vi "Lab Panel V4.90.vi"() -> ()   [LabVIEW 2013] (continued)
                    n844 = local read "SIG LAB04-1"() -> (w1524:T2)
                    n845 = stacked-sequence {
                      seq-local: [w1535 _] -> [_ w1539]
                      tunnel: w1533 -> [_ w1549]
                      tunnel: w1532 -> [_ w1548]
                      tunnel: w1531 -> [_ w1547]
                      tunnel: w1530 -> [_ w1546]
                      tunnel: w1529 -> [_ w1545]
                      tunnel: [_ w1544] -> w1528
                      tunnel: w1527 -> [_ w1543]
                      tunnel: w1526 -> [_ w1542]
                      tunnel: w1525 -> [_ w1541]
                      tunnel: w1524 -> [w1534 w1540]
                      tunnel: w1523 -> [_ w1538]
                      frame #0 {
                        n846 = Unbundle(w1534) -> ("AMPS"=w1537:dbl)  [unwired: 4 out]
                        n847 = call "Check For Amps on v1.vi"("ID"="LAB04-1", "amps"=w1537) -> ("amps"=w1535:bool)  [unwired: 9 in]
                      }
                      frame #1 {
                        n848 = case shown="True" w1539 {
                          tunnel: w1549 -> [_ w1562]
                          tunnel: w1548 -> [_ w1561]
                          tunnel: w1547 -> [_ w1560]
                          tunnel: w1546 -> [_ w1559]
                          tunnel: w1545 -> [_ w1558]
                          tunnel: [errorcluster {"status"=FALSE, "code"=0, "source"=""} ("error out") w1557] -> w1544
                          tunnel: w1543 -> [_ w1556]
                          tunnel: w1542 -> [_ w1555]
                          tunnel: w1541 -> [_ w1554]
                          tunnel: w1540 -> [_ w1553]
                          tunnel: w1538 -> [_ w1552]
                          frame False {
                            w1550 = FALSE
                            n849 = local write "RUN LAB04-1"(w1550) -> ()
                            n850 = local write "run lab04-1"(w1550) -> ()
                          }
                          frame True {
                            n851 = stacked-sequence {
                              seq-local: [w1563 _ _ _ _] -> [_ w1587 _ _ _]
                              tunnel: w1562 -> [w1568 _ _ _ _]
                              tunnel: w1561 -> [w1564 _ _ _ _]
                              tunnel: w1560 -> [w1578 _ _ _ _]
                              tunnel: w1559 -> [w1571 _ _ _ _]
                              tunnel: w1558 -> [w1566 _ _ _ _]
                              tunnel: [_ w1582 _ _ _] -> w1557
                              tunnel: w1556 -> [_ _ _ w1608 _]
                              tunnel: w1555 -> [_ _ _ w1607 _]
                              tunnel: w1554 -> [_ _ _ w1606 _]
                              tunnel: w1553 -> [_ _ _ _ _]
                              tunnel: w1552 -> [_ _ _ _ w1622]
                              frame #0 {
                                w1565 = "\\"
                                n852 = local read "SET LAB04-1"() -> (w1573:T5)
                                n853 = case shown="\"CYCLE TEST\"" w1578 {
                                tunnel: ["L04-1-CHART TEST-" "L04-1-CYCLE TEST-" "L04-1-T-RISE TEST-"] -> w1574
                                frame "CHART TEST", Default {
                                }
                                frame "CYCLE TEST" {
                                }
                                frame "T-RISE TEST" {
                                }
                                }
                                n854 = Unbundle(w1573) -> ("DESCRIPTION"=w1572:string)  [unwired: 4 out]
                                n855 = Concatenate Strings(w1568, "\\", w1566, w1565, w1564, w1565) -> (w1575:string)
                                n856 = String To Path(string=w1575) -> (path=w1577:path)
                                n857 = Concatenate Strings(w1575, w1574, w1572, "-", w1571, ".tdms") -> (w1563:string)
                                n858 = Create Folder(path (use dialog)=w1577) -> (error out=w1576:errorcluster)  [unwired: 2 in, 2 out]
                                n859 = global write "Global 1.vi" "LAB04-1 FILE"(w1563) -> ()
                                n860 = call <vilib>:"Clear Errors.vi"("error in (no error)"=w1576) -> ()  [unwired: 6 in, 1 out]
                              }
                              frame #1 {
                                (unwired) FALSE
                                n861 = String To Path(string=w1587) -> (path=w1583:path)
                                n862 = TDMS Open(6:FALSE, 10:T20."create or replace" ("operation (0:open)"), 11:w1583) -> (0:w1582:errorcluster, 3:→"TDMS LAB04-1":refnum<k34>)  [unwired: 4 in]
                              }
                              frame #2 {
                                n863 = local read "SET LAB04-1"() -> (w1593:T5)
                                n864 = local read "TDMS LAB04-1"() -> (w1604:refnum<k34>)
                                n865 = Build Array("Testers Name", "Description", "Set Test Cycles", "T-Rise minutes", "T-Rise Deg C") -> (w1594:string[])
                                n866 = Unbundle(w1593) -> ("NAME"=w1592:string, "DESCRIPTION"=w1591:string, "CYCLES"=w1590:dbl, "T-RISE mins"=w1589:dbl, "T-RISE deg C"=w1588:dbl)
                                n867 = Number To Decimal String(number=w1590) -> (decimal integer string=w1603:string)  [unwired: 1 in]
                                n868 = Number To Decimal String(number=w1589) -> (decimal integer string=w1602:string)  [unwired: 1 in]
                                n869 = Number To Decimal String(number=w1588) -> (decimal integer string=w1601:string)  [unwired: 1 in]
                                n870 = Build Array(w1592, w1591, w1603, w1602, w1601) -> (w1600:string[])
                                n871 = TDMS Set Properties(5:w1600, 7:w1594, 11:w1604) -> ()  [unwired: 3 in, 4 out]
                              }
                              frame #3 {
                                n872 = local read "DISP LAB04-1"() -> (w1609:T4)
                                n873 = Concatenate Strings("LAB04-1  ", w1608) -> (w1610:string)
                                n874 = Two Button Dialog(message=w1610, 1:w1606, 2:w1607) -> (T button?=w1612:bool)
                                n875 = case shown="True" w1612 {
                                tunnel: w1609 -> [w1619 w1620]
                                tunnel: [w1619 w1620] -> w1616
                                tunnel: [w1618 w1621] -> w1615
                                tunnel: [w1617 w1621] -> w1614
                                frame False {
                                n876 = Unbundle(w1619) -> ("CYCLE"=w1618:dbl, "MINS"=w1617:dbl)  [unwired: 1 out]
                                }
                                frame True {
                                w1621 = 0.0
                                }
                                }
                                n877 = Bundle(cluster=w1616, "CYCLE"=w1615, "MINS"=w1614, "STATUS"="RUN") -> (w1605:T4)
                                n878 = local write "DISP LAB04-1"(w1605) -> ()
                              }
                              frame #4 {
                                n879 = local read "TEMP START LAB04-1"() -> (w1624:cluster{"TL":dbl, "TN":dbl})
                                n880 = Bundle(cluster=w1624, "TL"=w1622, "TN"=w1622) -> (w1623:cluster{"TL":dbl, "TN":dbl})
                                n881 = local write "TEMP START LAB04-1"(w1623) -> ()
                              }
                            }
                          }
                        }
                      }
                    }
                  }
                }
              }
              event "RUN LAB04-2": Value Change {
                n882 = event-data() -> ("NewVal"=w1629:bool)  [unwired: 1 in, 5 out]
                n883 = local write "run lab04-2"(w1629) -> ()
                n884 = case shown="True" w1629 {
                  tunnel: w1635 -> [_ w1673]
                  tunnel: w1634 -> [_ w1672]
                  tunnel: w1632 -> [w1637 w1671]
                  tunnel: w1633 -> [_ w1670]
                  tunnel: w1631 -> [_ w1669]
                  tunnel: [w1636 w1668] -> w1630
                  tunnel: w1628 -> [_ w1667]
                  tunnel: w1627 -> [_ w1666]
                  tunnel: w1626 -> [_ w1665]
                  tunnel: w1625 -> [_ w1663]
                  frame False {
                    # "stop test"
                    n885 = stacked-sequence {
                      tunnel: w1637 -> [w1646 _]
                      tunnel: [w1638 _] -> w1636
                      frame #0 {
                        n886 = local read "DISP LAB04-2"() -> (w1645:T4)
                        n887 = Unbundle(w1645) -> ("CYCLE"=w1643:dbl, "MINS"=w1644:dbl)  [unwired: 1 out]
                        n888 = case shown="\"CYCLE TEST\"" w1646 {
                          tunnel: w1644 -> [_ _ w1653]
                          tunnel: w1643 -> [w1651 w1652 _]
                          tunnel: [w1651 w1652 w1653] -> w1642
                          frame "CHART TEST", Default {
                          }
                          frame "CYCLE TEST" {
                          }
                          frame "T-RISE TEST" {
                          }
                        }
                        n889 = local read "TDMS LAB04-2"() -> (w1650:refnum<k34>)
                        n890 = Build Array("STOPPED") -> (w1647:string[])
                        n891 = Build Array(w1642) -> (w1641:dbl[])
                        n892 = TDMS Write(0:w1650, 5:"TEST RESULT", 7:w1647, 9:w1641) -> (4:w1639:refnum<k34>, 15:w1640:errorcluster)  [unwired: 2 in, 2 out]
                        n893 = TDMS Close(8:w1640, 11:w1639) -> (0:w1638:errorcluster)  [unwired: 1 out]
                      }
                      frame #1 {
                        n894 = local read "DISP LAB04-2"() -> (w1657:T4)
                        n895 = stacked-sequence {
                          tunnel: "LAB04-2" -> [w1659 w1661]
                          frame #0 {
                            n896 = call "sub vi - defrag tdms v1.vi"("panel id"=w1659) -> ("error out"=w1658:errorcluster)  [unwired: 10 in]
                            n897 = local write "data file error"(w1658) -> ()
                          }
                          frame #1 {
                            n898 = call "Save data file (stop) v3.vi"("panel id"=w1661) -> ("network file save error"=w1660:errorcluster)  [unwired: 9 in, 1 out]
                            n899 = local write "RESULT LAB04-2"(FALSE) -> ()
                            n900 = local write "data file error"(w1660) -> ()
                          }
                        }
                        n901 = Bundle(cluster=w1657, "STATUS"="STOP") -> (w1655:T4)  [unwired: 2 in]
                        n902 = local write "DISP LAB04-2"(w1655) -> ()
                      }
                    }
                  }
                  frame True {
                    n903 = local read "SIG LAB04-2"() -> (w1664:T2)
                    n904 = stacked-sequence {
                      seq-local: [w1675 _] -> [_ w1679]
                      tunnel: w1673 -> [_ w1689]
                      tunnel: w1672 -> [_ w1688]
                      tunnel: w1671 -> [_ w1687]
                      tunnel: w1670 -> [_ w1686]
                      tunnel: w1669 -> [_ w1685]
                      tunnel: [_ w1684] -> w1668
                      tunnel: w1667 -> [_ w1683]
                      tunnel: w1666 -> [_ w1682]
                      tunnel: w1665 -> [_ w1681]
                      tunnel: w1664 -> [w1674 w1680]
                      tunnel: w1663 -> [_ w1678]
                      frame #0 {
                        n905 = Unbundle(w1674) -> ("AMPS"=w1677:dbl)  [unwired: 4 out]
                        n906 = call "Check For Amps on v1.vi"("ID"="LAB04-2", "amps"=w1677) -> ("amps"=w1675:bool)  [unwired: 9 in]
                      }
                      frame #1 {
                        n907 = case shown="True" w1679 {
                          tunnel: w1689 -> [_ w1702]
                          tunnel: w1688 -> [_ w1701]
                          tunnel: w1687 -> [_ w1700]
                          tunnel: w1686 -> [_ w1699]
                          tunnel: w1685 -> [_ w1698]
                          tunnel: [errorcluster {"status"=FALSE, "code"=0, "source"=""} ("error out") w1697] -> w1684
                          tunnel: w1683 -> [_ w1696]
                          tunnel: w1682 -> [_ w1695]
                          tunnel: w1681 -> [_ w1694]
                          tunnel: w1680 -> [_ w1693]
                          tunnel: w1678 -> [_ w1692]
                          frame False {
                            w1690 = FALSE
                            n908 = local write "RUN LAB04-2"(w1690) -> ()
                            n909 = local write "run lab04-2"(w1690) -> ()
                          }
                          frame True {
                            n910 = stacked-sequence {
                              seq-local: [w1703 _ _ _ _] -> [_ w1727 _ _ _]
                              tunnel: w1702 -> [w1708 _ _ _ _]
                              tunnel: w1701 -> [w1704 _ _ _ _]
                              tunnel: w1700 -> [w1718 _ _ _ _]
                              tunnel: w1699 -> [w1711 _ _ _ _]
                              tunnel: w1698 -> [w1706 _ _ _ _]
                              tunnel: [_ w1722 _ _ _] -> w1697
                              tunnel: w1696 -> [_ _ _ w1748 _]
                              tunnel: w1695 -> [_ _ _ w1747 _]
                              tunnel: w1694 -> [_ _ _ w1746 _]
                              tunnel: w1693 -> [_ _ _ _ _]
                              tunnel: w1692 -> [_ _ _ _ w1762]
                              frame #0 {
                                w1705 = "\\"
                                n911 = local read "SET LAB04-2"() -> (w1713:T5)
                                n912 = case shown="\"CHART TEST\", Default" w1718 {
                                tunnel: ["L04-2-CHART TEST-" "L04-2-CYCLE TEST-" "L04-2-T-RISE TEST-"] -> w1714
                                frame "CHART TEST", Default {
                                }
                                frame "CYCLE TEST" {
                                }
                                frame "T-RISE TEST" {
                                }
                                }
                                n913 = Unbundle(w1713) -> ("DESCRIPTION"=w1712:string)  [unwired: 4 out]
                                n914 = Concatenate Strings(w1708, "\\", w1706, w1705, w1704, w1705) -> (w1715:string)
                                n915 = String To Path(string=w1715) -> (path=w1717:path)
                                n916 = Concatenate Strings(w1715, w1714, w1712, "-", w1711, ".tdms") -> (w1703:string)
                                n917 = Create Folder(path (use dialog)=w1717) -> (error out=w1716:errorcluster)  [unwired: 2 in, 2 out]
                                n918 = global write "Global 1.vi" "LAB04-2 FILE"(w1703) -> ()
                                n919 = call <vilib>:"Clear Errors.vi"("error in (no error)"=w1716) -> ()  [unwired: 6 in, 1 out]
                              }
                              frame #1 {
                                (unwired) FALSE
                                n920 = String To Path(string=w1727) -> (path=w1723:path)
                                n921 = TDMS Open(6:FALSE, 10:T20."create or replace" ("operation (0:open)"), 11:w1723) -> (0:w1722:errorcluster, 3:→"TDMS LAB04-2":refnum<k34>)  [unwired: 4 in]
                              }
                              frame #2 {
                                n922 = local read "SET LAB04-2"() -> (w1733:T5)
                                n923 = local read "TDMS LAB04-2"() -> (w1744:refnum<k34>)
                                n924 = Build Array("Testers Name", "Description", "Set Test Cycles", "T-Rise minutes", "T-Rise Deg C") -> (w1734:string[])
                                n925 = Unbundle(w1733) -> ("NAME"=w1732:string, "DESCRIPTION"=w1731:string, "CYCLES"=w1730:dbl, "T-RISE mins"=w1729:dbl, "T-RISE deg C"=w1728:dbl)
                                n926 = Number To Decimal String(number=w1730) -> (decimal integer string=w1743:string)  [unwired: 1 in]
                                n927 = Number To Decimal String(number=w1729) -> (decimal integer string=w1742:string)  [unwired: 1 in]
                                n928 = Number To Decimal String(number=w1728) -> (decimal integer string=w1741:string)  [unwired: 1 in]
                                n929 = Build Array(w1732, w1731, w1743, w1742, w1741) -> (w1740:string[])
                                n930 = TDMS Set Properties(5:w1740, 7:w1734, 11:w1744) -> ()  [unwired: 3 in, 4 out]
                              }
                              frame #3 {
                                n931 = local read "DISP LAB04-2"() -> (w1749:T4)
                                n932 = Concatenate Strings("LAB04-2 ", w1748) -> (w1750:string)
                                n933 = Two Button Dialog(message=w1750, 1:w1746, 2:w1747) -> (T button?=w1752:bool)
                                n934 = case shown="True" w1752 {
                                tunnel: w1749 -> [w1759 w1760]
                                tunnel: [w1759 w1760] -> w1756
                                tunnel: [w1758 w1761] -> w1755
                                tunnel: [w1757 w1761] -> w1754
                                frame False {
                                n935 = Unbundle(w1759) -> ("CYCLE"=w1758:dbl, "MINS"=w1757:dbl)  [unwired: 1 out]
                                }
                                frame True {
                                w1761 = 0.0
                                }
                                }
                                n936 = Bundle(cluster=w1756, "CYCLE"=w1755, "MINS"=w1754, "STATUS"="RUN") -> (w1745:T4)
                                n937 = local write "DISP LAB04-2"(w1745) -> ()
                              }
                              frame #4 {
                                n938 = local read "TEMP START LAB04-2"() -> (w1764:cluster{"TL":dbl, "TN":dbl})
                                n939 = Bundle(cluster=w1764, "TL"=w1762, "TN"=w1762) -> (w1763:cluster{"TL":dbl, "TN":dbl})
                                n940 = local write "TEMP START LAB04-2"(w1763) -> ()
                              }
                            }
                          }
                        }
                      }
                    }
                  }
                }
              }
              event "RUN LAB05-1": Value Change {
                n941 = event-data() -> ("NewVal"=w1769:bool)  [unwired: 1 in, 5 out]
                n942 = local write "run lab05-1"(w1769) -> ()
                n943 = case shown="True" w1769 {
                  tunnel: w1775 -> [_ w1813]
                  tunnel: w1774 -> [_ w1812]
                  tunnel: w1772 -> [w1777 w1811]
                  tunnel: w1773 -> [_ w1810]
                  tunnel: w1771 -> [_ w1809]
                  tunnel: [w1776 w1808] -> w1770
                  tunnel: w1768 -> [_ w1807]
                  tunnel: w1767 -> [_ w1806]
                  tunnel: w1766 -> [_ w1805]
                  tunnel: w1765 -> [_ w1803]
                  frame False {
                    # "stop test"
                    n944 = stacked-sequence {
                      tunnel: w1777 -> [w1786 _]
                      tunnel: [w1778 _] -> w1776
                      frame #0 {
                        n945 = local read "DISP LAB05-1"() -> (w1785:T4)
                        n946 = Unbundle(w1785) -> ("CYCLE"=w1783:dbl, "MINS"=w1784:dbl)  [unwired: 1 out]
                        n947 = case shown="\"CYCLE TEST\"" w1786 {
                          tunnel: w1784 -> [_ _ w1793]
                          tunnel: w1783 -> [w1791 w1792 _]
                          tunnel: [w1791 w1792 w1793] -> w1782
                          frame "CHART TEST", Default {
                          }
                          frame "CYCLE TEST" {
                          }
                          frame "T-RISE TEST" {
                          }
                        }
                        n948 = local read "TDMS LAB05-1"() -> (w1790:refnum<k34>)
                        n949 = Build Array("STOPPED") -> (w1787:string[])
                        n950 = Build Array(w1782) -> (w1781:dbl[])
                        n951 = TDMS Write(0:w1790, 5:"TEST RESULT", 7:w1787, 9:w1781) -> (4:w1779:refnum<k34>, 15:w1780:errorcluster)  [unwired: 2 in, 2 out]
                        n952 = TDMS Close(8:w1780, 11:w1779) -> (0:w1778:errorcluster)  [unwired: 1 out]
                      }
                      frame #1 {
                        n953 = local read "DISP LAB05-1"() -> (w1797:T4)
                        n954 = stacked-sequence {
                          tunnel: "LAB05-1" -> [w1799 w1801]
                          frame #0 {
                            n955 = call "sub vi - defrag tdms v1.vi"("panel id"=w1799) -> ("error out"=w1798:errorcluster)  [unwired: 10 in]
                            n956 = local write "data file error"(w1798) -> ()
                          }
                          frame #1 {
                            n957 = call "Save data file (stop) v3.vi"("panel id"=w1801) -> ("network file save error"=w1800:errorcluster)  [unwired: 9 in, 1 out]
                            n958 = local write "RESULT LAB05-1"(FALSE) -> ()
                            n959 = local write "data file error"(w1800) -> ()
                          }
                        }
                        n960 = Bundle(cluster=w1797, "STATUS"="STOP") -> (w1795:T4)  [unwired: 2 in]
                        n961 = local write "DISP LAB05-1"(w1795) -> ()
                      }
                    }
                  }
                  frame True {
                    n962 = local read "SIG LAB05-1"() -> (w1804:T2)
                    n963 = stacked-sequence {
                      seq-local: [w1815 _] -> [_ w1819]
                      tunnel: w1813 -> [_ w1829]
                      tunnel: w1812 -> [_ w1828]
                      tunnel: w1811 -> [_ w1827]
                      tunnel: w1810 -> [_ w1826]
                      tunnel: w1809 -> [_ w1825]
                      tunnel: [_ w1824] -> w1808
                      tunnel: w1807 -> [_ w1823]
                      tunnel: w1806 -> [_ w1822]
                      tunnel: w1805 -> [_ w1821]
                      tunnel: w1804 -> [w1814 w1820]
                      tunnel: w1803 -> [_ w1818]
                      frame #0 {
                        n964 = Unbundle(w1814) -> ("AMPS"=w1817:dbl)  [unwired: 4 out]
                        n965 = call "Check For Amps on v1.vi"("ID"="LAB05-1", "amps"=w1817) -> ("amps"=w1815:bool)  [unwired: 9 in]
                      }
                      frame #1 {
                        n966 = case shown="True" w1819 {
                          tunnel: w1829 -> [_ w1842]
                          tunnel: w1828 -> [_ w1841]
                          tunnel: w1827 -> [_ w1840]
                          tunnel: w1826 -> [_ w1839]
                          tunnel: w1825 -> [_ w1838]
                          tunnel: [errorcluster {"status"=FALSE, "code"=0, "source"=""} ("error out") w1837] -> w1824
                          tunnel: w1823 -> [_ w1836]
                          tunnel: w1822 -> [_ w1835]
                          tunnel: w1821 -> [_ w1834]
                          tunnel: w1820 -> [_ w1833]
                          tunnel: w1818 -> [_ w1832]
                          frame False {
                            w1830 = FALSE
                            n967 = local write "RUN LAB05-1"(w1830) -> ()
                            n968 = local write "run lab05-1"(w1830) -> ()
                          }
                          frame True {
                            n969 = stacked-sequence {
                              seq-local: [w1843 _ _ _ _] -> [_ w1867 _ _ _]
                              tunnel: w1842 -> [w1848 _ _ _ _]
                              tunnel: w1841 -> [w1844 _ _ _ _]
                              tunnel: w1840 -> [w1858 _ _ _ _]
                              tunnel: w1839 -> [w1851 _ _ _ _]
                              tunnel: w1838 -> [w1846 _ _ _ _]
                              tunnel: [_ w1862 _ _ _] -> w1837
                              tunnel: w1836 -> [_ _ _ w1887 _]
                              tunnel: w1835 -> [_ _ _ w1886 _]
                              tunnel: w1834 -> [_ _ _ w1885 _]
                              tunnel: w1833 -> [_ _ _ _ _]
                              tunnel: w1832 -> [_ _ _ _ w1902]
                              frame #0 {
                                w1845 = "\\"
                                n970 = local read "SET LAB05-1"() -> (w1853:T5)
                                n971 = case shown="\"CYCLE TEST\"" w1858 {
                                tunnel: ["L05-1-CHART TEST-" "L05-1-CYCLE TEST-" "L05-1-T-RISE TEST-"] -> w1854
                                frame "CHART TEST", Default {
                                }
                                frame "CYCLE TEST" {
                                }
                                frame "T-RISE TEST" {
                                }
                                }
                                n972 = Unbundle(w1853) -> ("DESCRIPTION"=w1852:string)  [unwired: 4 out]
                                n973 = Concatenate Strings(w1848, "\\", w1846, w1845, w1844, w1845) -> (w1855:string)
                                n974 = String To Path(string=w1855) -> (path=w1857:path)
                                n975 = Concatenate Strings(w1855, w1854, w1852, "-", w1851, ".tdms") -> (w1843:string)
                                n976 = Create Folder(path (use dialog)=w1857) -> (error out=w1856:errorcluster)  [unwired: 2 in, 2 out]
                                n977 = global write "Global 1.vi" "LAB05-1 FILE"(w1843) -> ()
                                n978 = call <vilib>:"Clear Errors.vi"("error in (no error)"=w1856) -> ()  [unwired: 6 in, 1 out]
                              }
                              frame #1 {
                                (unwired) FALSE
                                n979 = String To Path(string=w1867) -> (path=w1863:path)
                                n980 = TDMS Open(6:FALSE, 10:T20."create or replace" ("operation (0:open)"), 11:w1863) -> (0:w1862:errorcluster, 3:→"TDMS LAB05-1":refnum<k34>)  [unwired: 4 in]
                              }
                              frame #2 {
                                n981 = local read "SET LAB05-1"() -> (w1873:T5)
                                n982 = local read "TDMS LAB05-1"() -> (w1884:refnum<k34>)
                                n983 = Build Array("Testers Name", "Description", "Set Test Cycles", "T-Rise minutes", "T-Rise Deg C") -> (w1874:string[])
                                n984 = Unbundle(w1873) -> ("NAME"=w1872:string, "DESCRIPTION"=w1871:string, "CYCLES"=w1870:dbl, "T-RISE mins"=w1869:dbl, "T-RISE deg C"=w1868:dbl)
                                n985 = Number To Decimal String(number=w1870) -> (decimal integer string=w1883:string)  [unwired: 1 in]
                                n986 = Number To Decimal String(number=w1869) -> (decimal integer string=w1882:string)  [unwired: 1 in]
                                n987 = Number To Decimal String(number=w1868) -> (decimal integer string=w1881:string)  [unwired: 1 in]
                                n988 = Build Array(w1872, w1871, w1883, w1882, w1881) -> (w1880:string[])
                                n989 = TDMS Set Properties(5:w1880, 7:w1874, 11:w1884) -> ()  [unwired: 3 in, 4 out]
                              }
                              frame #3 {
                                n990 = local read "DISP LAB05-1"() -> (w1889:T4)
                                n991 = Concatenate Strings("LAB05-1  ", w1887) -> (w1890:string)
                                n992 = Two Button Dialog(message=w1890, 1:w1885, 2:w1886) -> (T button?=w1892:bool)
                                n993 = case shown="True" w1892 {
                                tunnel: w1889 -> [w1899 w1900]
                                tunnel: [w1899 w1900] -> w1896
                                tunnel: [w1898 w1901] -> w1895
                                tunnel: [w1897 w1901] -> w1894
                                frame False {
                                n994 = Unbundle(w1899) -> ("CYCLE"=w1898:dbl, "MINS"=w1897:dbl)  [unwired: 1 out]
                                }
                                frame True {
                                w1901 = 0.0
                                }
                                }
                                n995 = Bundle(cluster=w1896, "CYCLE"=w1895, "MINS"=w1894, "STATUS"="RUN") -> (w1888:T4)
                                n996 = local write "DISP LAB05-1"(w1888) -> ()
                              }
                              frame #4 {
                                n997 = local read "TEMP START LAB05-1"() -> (w1904:cluster{"TL":dbl, "TN":dbl})
                                n998 = Bundle(cluster=w1904, "TL"=w1902, "TN"=w1902) -> (w1903:cluster{"TL":dbl, "TN":dbl})
                                n999 = local write "TEMP START LAB05-1"(w1903) -> ()
                              }
                            }
                          }
                        }
                      }
                    }
                  }
                }
              }
              event "RUN LAB05-2": Value Change {
                n1000 = event-data() -> ("NewVal"=w1910:bool)  [unwired: 1 in, 5 out]
                n1001 = local read "SIG LAB05-2"() -> (w1906:T2)
                n1002 = case shown="True" w1910 {
                  tunnel: w1916 -> [_ w1954]
                  tunnel: w1915 -> [_ w1953]
                  tunnel: w1913 -> [w1918 w1952]
                  tunnel: w1914 -> [_ w1951]
                  tunnel: w1912 -> [_ w1950]
                  tunnel: [w1917 w1949] -> w1911
                  tunnel: w1909 -> [_ w1948]
                  tunnel: w1908 -> [_ w1947]
                  tunnel: w1907 -> [_ w1946]
                  tunnel: w1906 -> [_ w1945]
                  tunnel: w1905 -> [_ w1944]
                  frame False {
                    # "stop test"
                    n1003 = stacked-sequence {
                      tunnel: w1918 -> [w1927 _]
                      tunnel: [w1919 _] -> w1917
                      frame #0 {
                        n1004 = local read "DISP LAB05-2"() -> (w1926:T4)
                        n1005 = Unbundle(w1926) -> ("CYCLE"=w1924:dbl, "MINS"=w1925:dbl)  [unwired: 1 out]
                        n1006 = case shown="\"CYCLE TEST\"" w1927 {
                          tunnel: w1925 -> [_ _ w1934]
                          tunnel: w1924 -> [w1932 w1933 _]
                          tunnel: [w1932 w1933 w1934] -> w1923
                          frame "CHART TEST", Default {
                          }
                          frame "CYCLE TEST" {
                          }
                          frame "T-RISE TEST" {
                          }
                        }
                        n1007 = local read "TDMS LAB05-2"() -> (w1931:refnum<k34>)
                        n1008 = Build Array("STOPPED") -> (w1928:string[])
                        n1009 = Build Array(w1923) -> (w1922:dbl[])
                        n1010 = TDMS Write(0:w1931, 5:"TEST RESULT", 7:w1928, 9:w1922) -> (4:w1920:refnum<k34>, 15:w1921:errorcluster)  [unwired: 2 in, 2 out]
                        n1011 = TDMS Close(8:w1921, 11:w1920) -> (0:w1919:errorcluster)  [unwired: 1 out]
                      }
                      frame #1 {
                        n1012 = local read "DISP LAB05-2"() -> (w1938:T4)
                        n1013 = stacked-sequence {
                          tunnel: "LAB05-2" -> [w1940 w1942]
                          frame #0 {
                            n1014 = call "sub vi - defrag tdms v1.vi"("panel id"=w1940) -> ("error out"=w1939:errorcluster)  [unwired: 10 in]
                            n1015 = local write "data file error"(w1939) -> ()
                          }
                          frame #1 {
                            n1016 = local write "RESULT LAB05-2"(FALSE) -> ()
                            n1017 = call "Save data file (stop) v3.vi"("panel id"=w1942) -> ("network file save error"=w1941:errorcluster)  [unwired: 9 in, 1 out]
                            n1018 = local write "data file error"(w1941) -> ()
                          }
                        }
                        n1019 = Bundle(cluster=w1938, "STATUS"="STOP") -> (w1936:T4)  [unwired: 2 in]
                        n1020 = local write "DISP LAB05-2"(w1936) -> ()
                      }
                    }
                  }
                  frame True {
                    n1021 = stacked-sequence {
                      seq-local: [w1956 _] -> [_ w1960]
                      tunnel: w1954 -> [_ w1970]
                      tunnel: w1953 -> [_ w1969]
                      tunnel: w1952 -> [_ w1968]
                      tunnel: w1951 -> [_ w1967]
                      tunnel: w1950 -> [_ w1966]
                      tunnel: [_ w1965] -> w1949
                      tunnel: w1948 -> [_ w1964]
                      tunnel: w1947 -> [_ w1963]
                      tunnel: w1946 -> [_ w1962]
                      tunnel: w1945 -> [w1955 w1961]
                      tunnel: w1944 -> [_ w1959]
                      frame #0 {
                        n1022 = Unbundle(w1955) -> ("AMPS"=w1958:dbl)  [unwired: 4 out]
                        n1023 = call "Check For Amps on v1.vi"("ID"="LAB05-2", "amps"=w1958) -> ("amps"=w1956:bool)  [unwired: 9 in]
                      }
                      frame #1 {
                        n1024 = case shown="True" w1960 {
                          tunnel: w1970 -> [_ w1983]
                          tunnel: w1969 -> [_ w1982]
                          tunnel: w1968 -> [_ w1981]
                          tunnel: w1967 -> [_ w1980]
                          tunnel: w1966 -> [_ w1979]
                          tunnel: [errorcluster {"status"=FALSE, "code"=0, "source"=""} ("error out") w1978] -> w1965
                          tunnel: w1964 -> [_ w1977]
                          tunnel: w1963 -> [_ w1976]
                          tunnel: w1962 -> [_ w1975]
                          tunnel: w1961 -> [_ w1974]
                          tunnel: w1959 -> [_ w1973]
                          frame False {
                            w1971 = FALSE
                            n1025 = local write "RUN LAB05-2"(w1971) -> ()
                            n1026 = local write "run lab05-2"(w1971) -> ()
                          }
                          frame True {
                            n1027 = stacked-sequence {
                              seq-local: [w1984 _ _ _ _] -> [_ w2008 _ _ _]
                              tunnel: w1983 -> [w1989 _ _ _ _]
                              tunnel: w1982 -> [w1985 _ _ _ _]
                              tunnel: w1981 -> [w1999 _ _ _ _]
                              tunnel: w1980 -> [w1992 _ _ _ _]
                              tunnel: w1979 -> [w1987 _ _ _ _]
                              tunnel: [_ w2003 _ _ _] -> w1978
                              tunnel: w1977 -> [_ _ _ w2028 _]
                              tunnel: w1976 -> [_ _ _ w2027 _]
                              tunnel: w1975 -> [_ _ _ w2026 _]
                              tunnel: w1974 -> [_ _ _ _ _]
                              tunnel: w1973 -> [_ _ _ _ w2043]
                              frame #0 {
                                w1986 = "\\"
                                n1028 = local read "SET LAB05-2"() -> (w1994:T5)
                                n1029 = case shown="\"CYCLE TEST\"" w1999 {
                                tunnel: ["L05-2-CHART TEST-" "L05-2-CYCLE TEST-" "L05-2-T-RISE TEST-"] -> w1995
                                frame "CHART TEST", Default {
                                }
                                frame "CYCLE TEST" {
                                }
                                frame "T-RISE TEST" {
                                }
                                }
                                n1030 = Unbundle(w1994) -> ("DESCRIPTION"=w1993:string)  [unwired: 4 out]
                                n1031 = Concatenate Strings(w1989, "\\", w1987, w1986, w1985, w1986) -> (w1996:string)
                                n1032 = String To Path(string=w1996) -> (path=w1998:path)
                                n1033 = Concatenate Strings(w1996, w1995, w1993, "-", w1992, ".tdms") -> (w1984:string)
                                n1034 = Create Folder(path (use dialog)=w1998) -> (error out=w1997:errorcluster)  [unwired: 2 in, 2 out]
                                n1035 = global write "Global 1.vi" "LAB05-2 FILE"(w1984) -> ()
                                n1036 = call <vilib>:"Clear Errors.vi"("error in (no error)"=w1997) -> ()  [unwired: 6 in, 1 out]
                              }
                              frame #1 {
                                (unwired) FALSE
                                n1037 = String To Path(string=w2008) -> (path=w2004:path)
                                n1038 = TDMS Open(6:FALSE, 10:T20."create or replace" ("operation (0:open)"), 11:w2004) -> (0:w2003:errorcluster, 3:→"TDMS LAB05-2":refnum<k34>)  [unwired: 4 in]
                              }
                              frame #2 {
                                n1039 = local read "SET LAB05-2"() -> (w2014:T5)
                                n1040 = local read "TDMS LAB05-2"() -> (w2025:refnum<k34>)
                                n1041 = Build Array("Testers Name", "Description", "Set Test Cycles", "T-Rise minutes", "T-Rise Deg C") -> (w2015:string[])
                                n1042 = Unbundle(w2014) -> ("NAME"=w2013:string, "DESCRIPTION"=w2012:string, "CYCLES"=w2011:dbl, "T-RISE mins"=w2010:dbl, "T-RISE deg C"=w2009:dbl)
                                n1043 = Number To Decimal String(number=w2011) -> (decimal integer string=w2024:string)  [unwired: 1 in]
                                n1044 = Number To Decimal String(number=w2010) -> (decimal integer string=w2023:string)  [unwired: 1 in]
                                n1045 = Number To Decimal String(number=w2009) -> (decimal integer string=w2022:string)  [unwired: 1 in]
                                n1046 = Build Array(w2013, w2012, w2024, w2023, w2022) -> (w2021:string[])
                                n1047 = TDMS Set Properties(5:w2021, 7:w2015, 11:w2025) -> ()  [unwired: 3 in, 4 out]
                              }
                              frame #3 {
                                n1048 = local read "DISP LAB05-2"() -> (w2030:T4)
                                n1049 = Concatenate Strings("LAB05-2  ", w2028) -> (w2031:string)
                                n1050 = Two Button Dialog(message=w2031, 1:w2026, 2:w2027) -> (T button?=w2033:bool)
                                n1051 = case shown="True" w2033 {
                                tunnel: w2030 -> [w2040 w2041]
                                tunnel: [w2040 w2041] -> w2037
                                tunnel: [w2039 w2042] -> w2036
                                tunnel: [w2038 w2042] -> w2035
                                frame False {
                                n1052 = Unbundle(w2040) -> ("CYCLE"=w2039:dbl, "MINS"=w2038:dbl)  [unwired: 1 out]
                                }
                                frame True {
                                w2042 = 0.0
                                }
                                }
                                n1053 = Bundle(cluster=w2037, "CYCLE"=w2036, "MINS"=w2035, "STATUS"="RUN") -> (w2029:T4)
                                n1054 = local write "DISP LAB05-2"(w2029) -> ()
                              }
                              frame #4 {
                                n1055 = local read "TEMP START LAB05-2"() -> (w2045:cluster{"TL":dbl, "TN":dbl})
                                n1056 = Bundle(cluster=w2045, "TL"=w2043, "TN"=w2043) -> (w2044:cluster{"TL":dbl, "TN":dbl})
                                n1057 = local write "TEMP START LAB05-2"(w2044) -> ()
                              }
                            }
                          }
                        }
                      }
                    }
                  }
                }
                n1058 = local write "run lab05-2"(w1910) -> ()
              }
            }
            n1059 = local write "data file error"(w614) -> ()
          }
          frame #4 {
            # "check if test cycles reached for cycle tests, if so then test pass"
            n1060 = stacked-sequence {
              tunnel: w2065 -> [_ _ _ _ _ _ _ _ _ _]
              tunnel: w2064 -> [_ _ _ _ _ _ _ _ _ _]
              tunnel: w2063 -> [_ _ _ _ _ _ _ _ _ _]
              tunnel: w2062 -> [_ _ _ _ _ _ _ _ _ _]
              tunnel: w2061 -> [_ _ _ _ _ _ _ _ _ _]
              tunnel: w2060 -> [_ _ _ _ _ _ _ _ _ _]
              tunnel: w2059 -> [_ _ _ _ _ _ _ _ _ _]
              tunnel: w2058 -> [_ _ _ _ _ _ _ _ _ _]
              tunnel: w2057 -> [_ _ _ _ _ _ _ _ _ _]
              tunnel: w2056 -> [_ _ _ _ _ _ _ _ _ _]
              tunnel: w2055 -> [w2071 _ _ _ _ _ _ _ _ _]
              tunnel: w2054 -> [_ w2106 _ _ _ _ _ _ _ _]
              tunnel: w2053 -> [_ _ w2146 _ _ _ _ _ _ _]
              tunnel: w2052 -> [_ _ _ w2186 _ _ _ _ _ _]
              tunnel: w2051 -> [_ _ _ _ w2226 _ _ _ _ _]
              tunnel: w2050 -> [_ _ _ _ _ w2266 _ _ _ _]
              tunnel: w2049 -> [_ _ _ _ _ _ w2306 _ _ _]
              tunnel: w2048 -> [_ _ _ _ _ _ _ w2346 _ _]
              tunnel: w2047 -> [_ _ _ _ _ _ _ _ w2386 _]
              tunnel: w2046 -> [_ _ _ _ _ _ _ _ _ w2426]
              frame #0 {
                # "LAB01-1"
                n1061 = Less?(x=w2071, y=2) -> (x < y?=w2069:bool)
                n1062 = local read "DISP LAB01-1"() -> (w2072:T4)
                n1063 = Unbundle(w2072) -> ("STATUS"=w2066:string)  [unwired: 2 out]
                n1064 = Equal?(x=w2066, y="RUN") -> (x = y?=w2068:bool)
                n1065 = And(x=w2068, y=w2069) -> (x .and. y?=w2067:bool)
                n1066 = case shown="True" w2067 {
                  tunnel: w2072 -> [_ w2077]
                  tunnel: w2071 -> [_ w2081]
                  frame False {
                  }
                  frame True {
                    n1067 = local read "SET LAB01-1"() -> (w2083:T5)
                    n1068 = local read "TDMS LAB01-1"() -> (w2076:refnum<k34>)
                    n1069 = Unbundle(w2083) -> ("CYCLES"=w2074:dbl, "T-RISE mins"=w2080:dbl)  [unwired: 3 out]
                    n1070 = case shown="\"CYCLE TEST\"" w2081 {
                      tunnel: w2080 -> [_ _ w2090]
                      tunnel: [w2085 w2087 w2090] -> w2079
                      tunnel: w2074 -> [w2085 w2087 _]
                      tunnel: ["CHART PASS" "CYCLE PASS" "T-RISE PASS"] -> w2078
                      frame "CHART TEST", Default {
                      }
                      frame "CYCLE TEST" {
                      }
                      frame "T-RISE TEST" {
                      }
                    }
                    n1071 = Unbundle(w2077) -> ("CYCLE"=w2082:dbl)  [unwired: 2 out]
                    n1072 = Increment(x=w2074) -> (x+1=w2075:dbl)
                    n1073 = Greater Or Equal?(x=w2082, y=w2075) -> (x >= y?=w2084:bool)
                    n1074 = case shown="True" w2084 {
                      tunnel: w2079 -> [w2094 _]
                      tunnel: w2078 -> [w2093 _]
                      tunnel: w2077 -> [w2092 _]
                      tunnel: w2076 -> [w2091 _]
                      frame True {
                        n1075 = stacked-sequence {
                          tunnel: w2094 -> [w2098 _]
                          tunnel: w2093 -> [w2096 w2102]
                          tunnel: w2092 -> [_ w2105]
                          tunnel: w2091 -> [w2095 _]
                          frame #0 {
                            n1076 = Build Array(w2096) -> (w2099:string[])
                            n1077 = Build Array(w2098) -> (w2097:dbl[])
                            n1078 = TDMS Write(0:w2095, 5:"TEST PASS", 7:w2099, 9:w2097) -> (15:w2101:errorcluster)  [unwired: 2 in, 3 out]
                            n1079 = local write "data file error"(w2101) -> ()
                          }
                          frame #1 {
                            n1080 = Bundle(cluster=w2105, "STATUS"=w2102) -> (w2103:T4)  [unwired: 2 in]
                            n1081 = local write "RESULT LAB01-1"(TRUE) -> ()
                            n1082 = local write "DISP LAB01-1"(w2103) -> ()
                          }
                        }
                      }
                      frame False {
                      }
                    }
                  }
                }
              }
              frame #1 {
                # "LAB01-2"
                n1083 = Less?(x=w2106, y=2) -> (x < y?=w2109:bool)
                n1084 = local read "DISP LAB01-2"() -> (w2111:T4)
                n1085 = Unbundle(w2111) -> ("STATUS"=w2112:string)  [unwired: 2 out]
                n1086 = Equal?(x=w2112, y="RUN") -> (x = y?=w2108:bool)
                n1087 = And(x=w2108, y=w2109) -> (x .and. y?=w2107:bool)
                n1088 = case shown="True" w2107 {
                  tunnel: w2111 -> [_ w2117]
                  tunnel: w2106 -> [_ w2121]
                  frame False {
                  }
                  frame True {
                    n1089 = local read "SET LAB01-2"() -> (w2123:T5)
                    n1090 = local read "TDMS LAB01-2"() -> (w2116:refnum<k34>)
                    n1091 = Unbundle(w2123) -> ("CYCLES"=w2114:dbl, "T-RISE mins"=w2120:dbl)  [unwired: 3 out]
                    n1092 = case shown="\"T-RISE TEST\"" w2121 {
                      tunnel: w2120 -> [_ _ w2130]
                      tunnel: [w2125 w2127 w2130] -> w2119
                      tunnel: w2114 -> [w2125 w2127 _]
                      tunnel: ["CHART PASS" "CYCLE PASS" "T-RISE PASS"] -> w2118
                      frame "CHART TEST", Default {
                      }
                      frame "CYCLE TEST" {
                      }
                      frame "T-RISE TEST" {
                      }
                    }
                    n1093 = Unbundle(w2117) -> ("CYCLE"=w2122:dbl)  [unwired: 2 out]
                    n1094 = Increment(x=w2114) -> (x+1=w2115:dbl)
                    n1095 = Greater Or Equal?(x=w2122, y=w2115) -> (x >= y?=w2124:bool)
                    n1096 = case shown="True" w2124 {
                      tunnel: w2119 -> [w2134 _]
                      tunnel: w2118 -> [w2133 _]
                      tunnel: w2117 -> [w2132 _]
                      tunnel: w2116 -> [w2131 _]
                      frame True {
                        n1097 = stacked-sequence {
                          tunnel: w2134 -> [w2138 _]
                          tunnel: w2133 -> [w2136 w2142]
                          tunnel: w2132 -> [_ w2145]
                          tunnel: w2131 -> [w2135 _]
                          frame #0 {
                            n1098 = Build Array(w2136) -> (w2139:string[])
                            n1099 = Build Array(w2138) -> (w2137:dbl[])
                            n1100 = TDMS Write(0:w2135, 5:"TEST PASS", 7:w2139, 9:w2137) -> (15:w2141:errorcluster)  [unwired: 2 in, 3 out]
                            n1101 = local write "data file error"(w2141) -> ()
                          }
                          frame #1 {
                            n1102 = Bundle(cluster=w2145, "STATUS"=w2142) -> (w2143:T4)  [unwired: 2 in]
                            n1103 = local write "RESULT LAB01-2"(TRUE) -> ()
                            n1104 = local write "DISP LAB01-2"(w2143) -> ()
                          }
                        }
                      }
                      frame False {
                      }
                    }
                  }
                }
              }
              frame #2 {
                # "LAB02-1"
                n1105 = Less?(x=w2146, y=2) -> (x < y?=w2149:bool)
                n1106 = local read "DISP LAB02-1"() -> (w2151:T4)
                n1107 = Unbundle(w2151) -> ("STATUS"=w2152:string)  [unwired: 2 out]
                n1108 = Equal?(x=w2152, y="RUN") -> (x = y?=w2148:bool)
                n1109 = And(x=w2148, y=w2149) -> (x .and. y?=w2147:bool)
                n1110 = case shown="True" w2147 {
                  tunnel: w2151 -> [_ w2157]
                  tunnel: w2146 -> [_ w2161]
                  frame False {
                  }
                  frame True {
                    n1111 = local read "SET LAB02-1"() -> (w2163:T5)
                    n1112 = local read "TDMS LAB02-1"() -> (w2156:refnum<k34>)
                    n1113 = Unbundle(w2157) -> ("CYCLE"=w2162:dbl)  [unwired: 2 out]
                    n1114 = Unbundle(w2163) -> ("CYCLES"=w2154:dbl, "T-RISE mins"=w2160:dbl)  [unwired: 3 out]
                    n1115 = case shown="\"T-RISE TEST\"" w2161 {
                      tunnel: w2160 -> [_ _ w2170]
                      tunnel: [w2165 w2167 w2170] -> w2159
                      tunnel: w2154 -> [w2165 w2167 _]
                      tunnel: ["CHART PASS" "CYCLE PASS" "T-RISE PASS"] -> w2158
                      frame "CHART TEST", Default {
                      }
                      frame "CYCLE TEST" {
                      }
                      frame "T-RISE TEST" {
                      }
                    }
                    n1116 = Increment(x=w2154) -> (x+1=w2155:dbl)
